vi "Example.vi"() -> ()   [LabVIEW 2017, in "Basic Example.lvlib"]
uses:
  Basic Example.lvlib
  Promise Future/Future/Future.lvclass/Future.ctl
  2841eb21-99c0-4648-9142-7390a639aaf0.vi
  2051c695-3874-48ea-ae31-7f745d14b586.vi
  8bb1566a-2ed5-428d-ab5d-8d91b9f93975.vi
  c7557200-e4cb-4974-b6a7-c6446bd508d1.vi
  76060e51-b76b-4b50-a505-5a03475d9830.vi
  Promise Future/Future/Then.vi
  Promise Future/Promise/Promise.lvclass
  E:/Promise/Promise Future/Future/Future.lvclass
  Promise Future/Promise/Read Future.vi
  Promise Future/Future/Read Value (private).vi
  Promise Future/Future/Fulfull (Value).vi
  Promise Future/Future/VI Name Wrapper.vi
  Promise Future/State/Then.vi
  <vilib>/Utility/error.llb/Error Cluster From Error Code.vi
  Promise Future/Future/Future.lvclass
  <vilib>/ErrorRing/Error Ring.xnode
panel:
  in  "Scope":string
  out "Value":string
  in  "Then Button":bool
  in  "Value":string
  in  "Set Button":bool
  out "Value 2":string
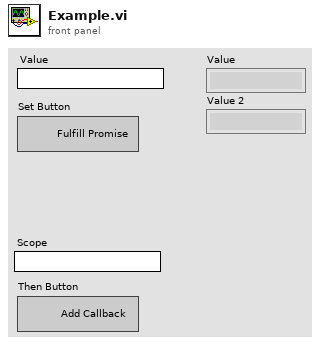
[diagram p1: front panel]
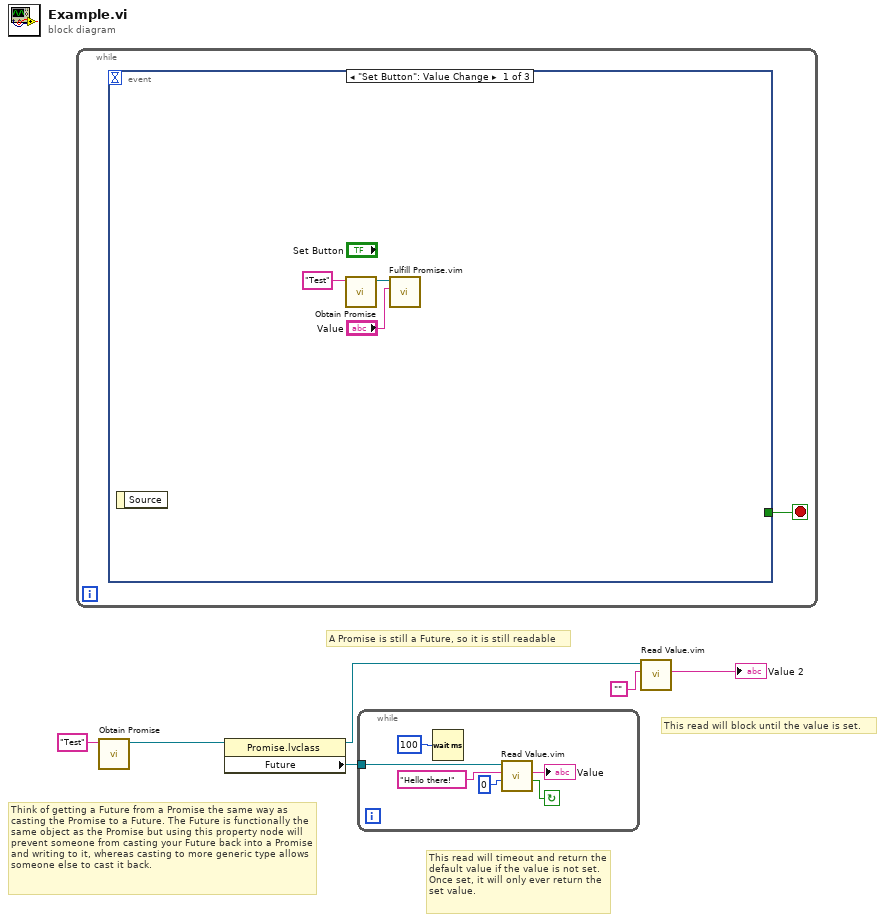
[diagram p0: block diagram]
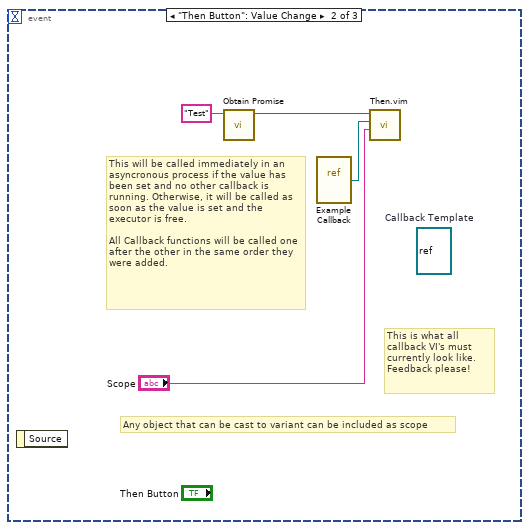
[diagram p2: hidden frame]
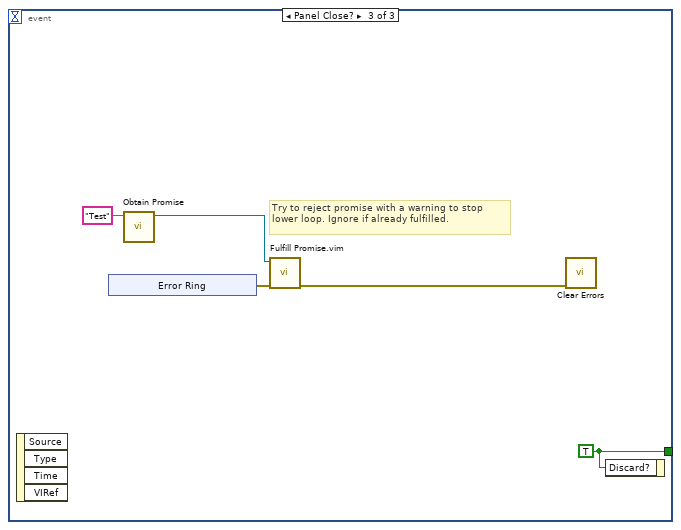
[diagram p3: hidden frame]
diagram:
  # "This read will timeout and return the default value if the value is not set. Once set, it will only ever return the set value."
  # "This read will block until the value is set."
  # "Think of getting a Future from a Promise the same way as casting the Promise to a Future. The Future is functionally the same object as the Promise but using this property node will prevent someone from casting your Future back into a Promise and writing to it, whereas casting to more generic type allows someone else to cast it back."
  # "A Promise is still a Future, so it is still readable"
  n1 = while {
    stop <- w7 stop-if-true
    n2 = event shown="[0] \"Set Button\": Value Change" {
      selector: _ -> [_ _ _]
      dyn-events: _ -> [_ _ _]
      timeout: _ -> [_ _ _]
      tunnel: [_ _ w17] -> w7
      event "Set Button": Value Change {
        n3 = event-data() -> ()  [unwired: 1 in, 1 out]
        n4 = call "Obtain Promise.vi"("name (unnamed)"="Test") -> ("Promise out"=w8:refnum<class "Promise.lvclass">)  [unwired: 8 in, 2 out]
        n5 = call "Fulfill Promise.vim"("Value"="Value", "Promise in"=w8) -> ()  [unwired: 8 in, 2 out]
      }
      event "Then Button": Value Change {
        (unwired) refnum<vi> refnum  # Callback Template
        # "Any object that can be cast to variant can be included as scope"
        # "This is what all callback VI's must currently look like. Feedback please!"
        # "This will be called immediately in an asyncronous process if the value has been set and no other callback is running. Otherwise, it will be called as soon as the value is set and the executor is free.\n\nAll Callback functions will be called one after the other in the same order they were added."
        n6 = event-data() -> ()  [unwired: 1 in, 1 out]
        n7 = call "Obtain Promise.vi"("name (unnamed)"="Test") -> ("Promise out"=w11:refnum<class "Promise.lvclass">)  [unwired: 8 in, 2 out]
        n8 = vi-ref "Example Callback.vi"() -> (w14:refnum<vi>)
        n9 = call "Then.vim"("Scope"="Scope", "Callback"=w14, "Future in"=w11) -> ()  [unwired: 7 in, 2 out]
      }
      event Panel Close? {
        w17 = TRUE ("Discard?")
        # "Try to reject promise with a warning to stop lower loop. Ignore if already fulfilled."
        n10 = event-data() -> ()  [unwired: 1 in, 4 out]
        n11 = xnode "Error Ring"() -> ("error out"=w15:errorcluster)
        n12 = call "Obtain Promise.vi"("name (unnamed)"="Test") -> ("Promise out"=w18:refnum<class "Promise.lvclass">)  [unwired: 8 in, 2 out]
        n13 = call "Fulfill Promise.vim"("error in (no error)"=w15, "Promise in"=w18) -> ("error out"=w16:errorcluster)  [unwired: 8 in, 1 out]
        n14 = call <vilib>:"Clear Errors.vi"("error in (no error)"=w16) -> ()  [unwired: 5 in, 2 out]
        n15 = event-data("Discard?"=w17) -> ()  [unwired: 1 in, 1 out]
      }
    }
  }
  n16 = call "Obtain Promise.vi"("name (unnamed)"="Test") -> ("Promise out"=w1:refnum<class "Promise.lvclass">)  [unwired: 8 in, 2 out]
  n17 = property class="Promise.lvclass"(reference=w1) -> (reference out=w2:refnum<class "Promise.lvclass">, "Future"=w4:refnum<class "Future.lvclass">)  [unwired: 1 in, 1 out]
  n18 = while {
    tunnel: w4 -> [w26]
    stop <- w25 continue-if-true
    n19 = Wait (ms)(milliseconds to wait=u32 100) -> ()  [unwired: 1 out]
    n20 = call "Read Value.vim"("timeout in ms (-1)"=0, "Default Value"="Hello there!", "Future in"=w26) -> ("timed out?"=w25:bool, "Value"=→"Value":string)  [unwired: 5 in, 2 out]
  }
  n21 = call "Read Value.vim"("Default Value"="", "Future in"=w2) -> ("Value"=→"Value 2":string)  [unwired: 6 in, 3 out]
